vi "Exercise 10.3_Answer.vi"() -> ()   [LabVIEW 2010]
uses:
  Global 1.vi
panel:
  in  "Restart":bool
  in  "Stop":bool
  in  "Walk Request":bool
  out "Walk Sign":bool
  out "Green":bool
  out "Yellow":bool
  out "Red":bool
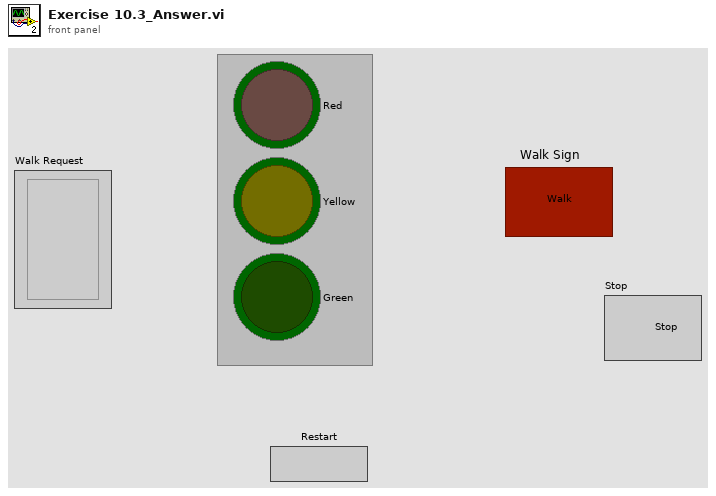
[diagram p1: front panel]
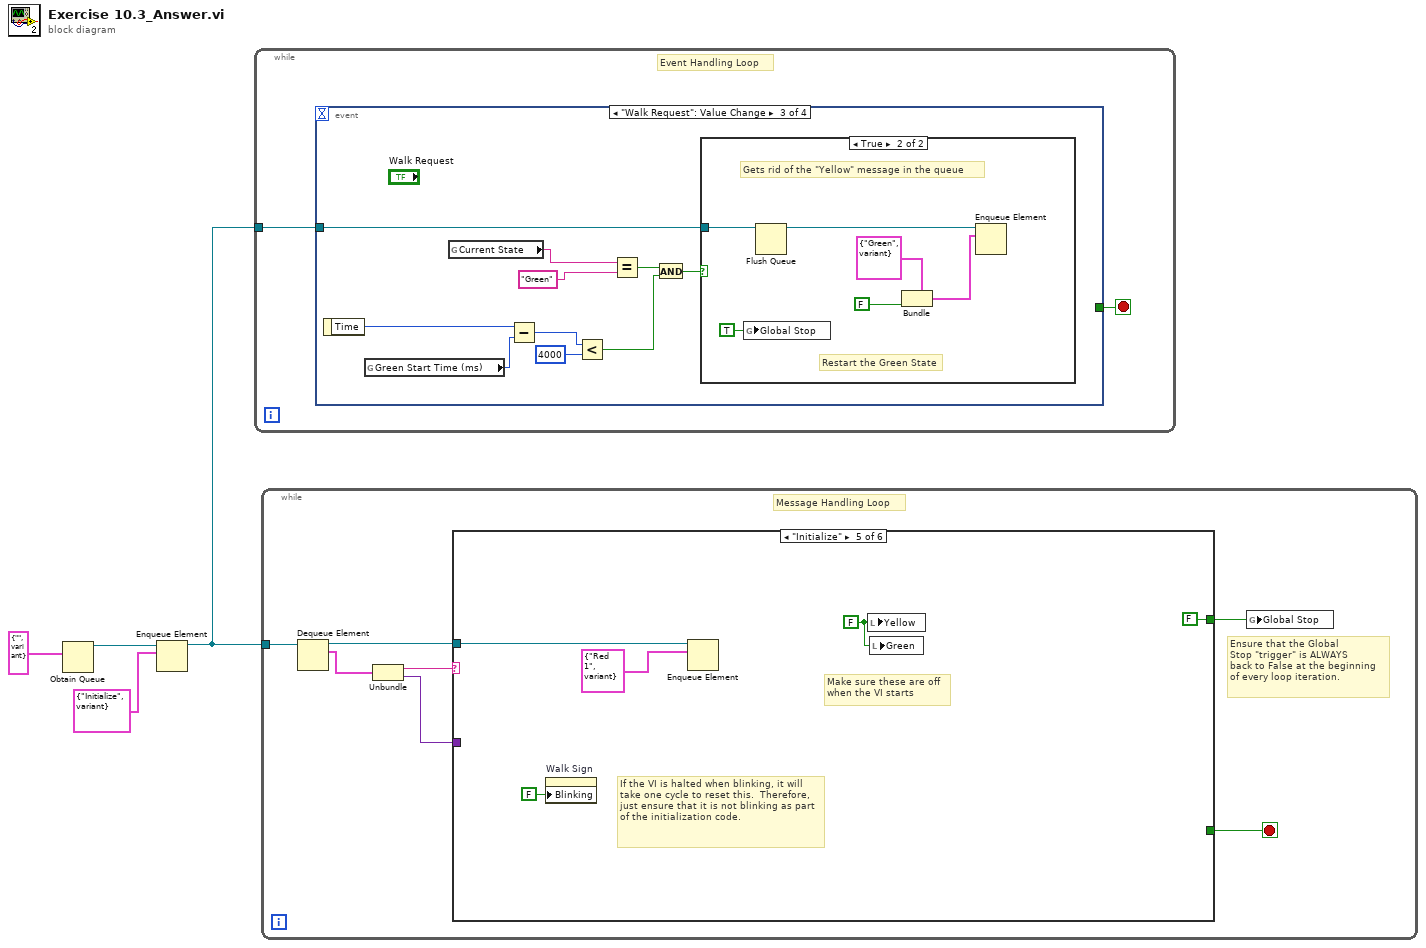
[diagram p0: block diagram]
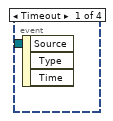
[diagram p2: hidden frame]
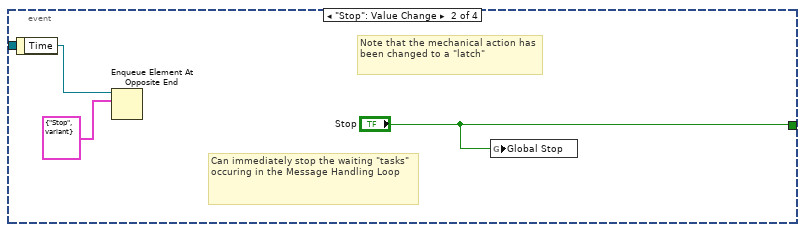
[diagram p3: hidden frame]
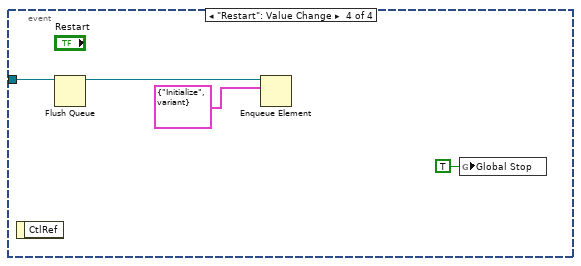
[diagram p5: hidden frame]
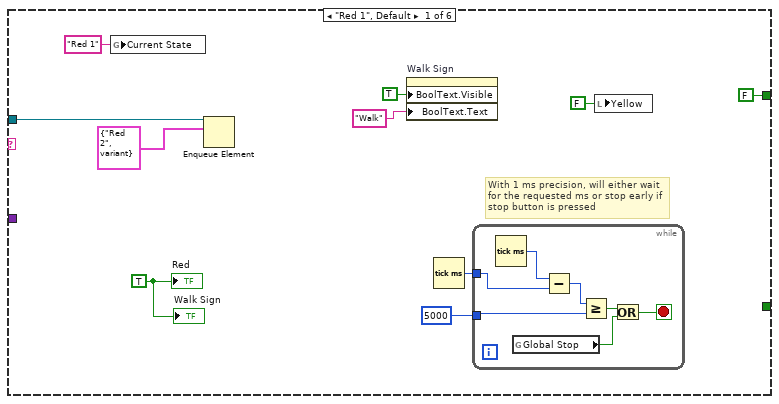
[diagram p6: hidden frame]
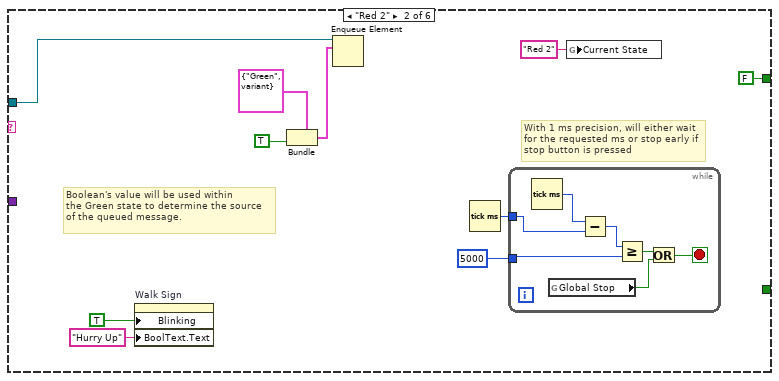
[diagram p7: hidden frame]
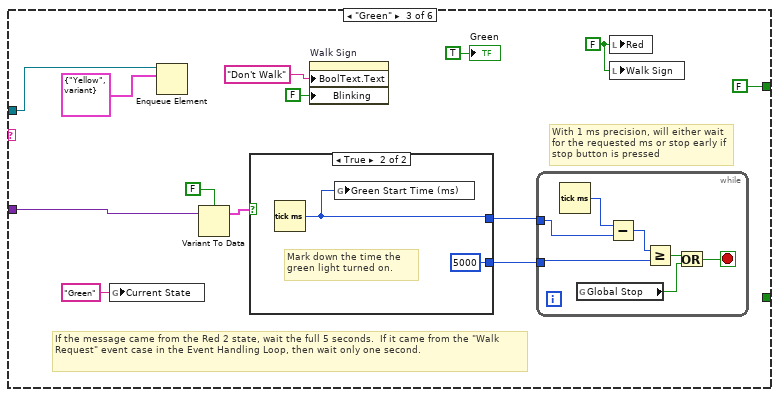
[diagram p8: hidden frame]
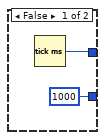
[diagram p9: hidden frame]
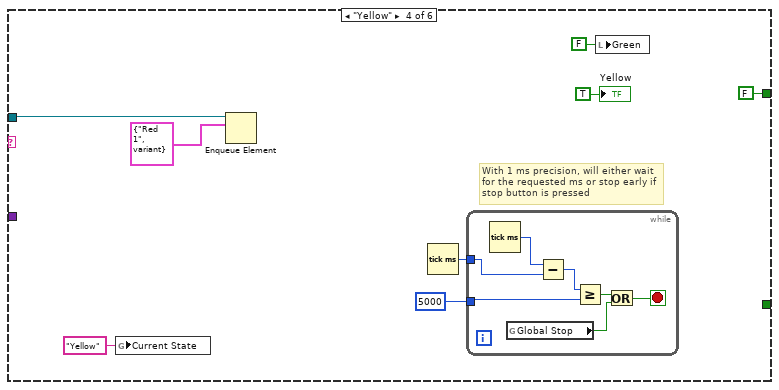
[diagram p10: hidden frame]
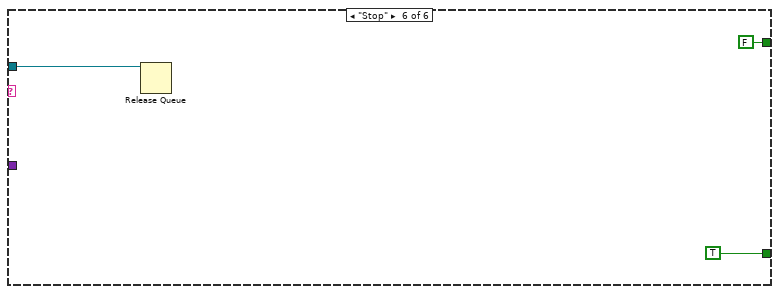
[diagram p11: hidden frame]
diagram:
  n1 = Obtain Queue(element data type=cluster{string, variant} {"", variant}) -> (queue out=w3:refnum<queue>)  [unwired: 4 in, 2 out]
  n2 = Enqueue Element(queue=w3, element=cluster{string, variant} {"Initialize", variant}) -> (queue out=w1:refnum<queue>)  [unwired: 2 in, 2 out]
  n3 = while {
    tunnel: w1 -> [w5]
    stop <- w6 stop-if-true
    # "Event Handling Loop"
    n4 = event shown="[2] \"Walk Request\": Value Change" {
      selector: _ -> [_ _ _ _]
      dyn-events: _ -> [_ _ _ _]
      timeout: _ -> [_ _ _ _]
      tunnel: [_ "Stop" _ _] -> w6
      tunnel: w5 -> [_ w8 w11 w27]
      event Timeout {
        n5 = event-data() -> ()  [unwired: 1 in, 3 out]
      }
      event "Stop": Value Change {
        # "Can immediately stop the waiting \"tasks\" occuring in the Message Handling Loop"
        # "Note that the mechanical action has been changed to a \"latch\""
        n6 = event-data() -> ()  [unwired: 1 in, 1 out]
        n7 = Enqueue Element At Opposite End(queue=w8, element=cluster{string, variant} {"Stop", variant}) -> ()  [unwired: 2 in, 3 out]
        n8 = global write "Global 1.vi" "Global Stop"("Stop") -> ()
      }
      event "Walk Request": Value Change {
        n9 = event-data() -> ("Time"=w19:u32)  [unwired: 1 in]
        n10 = global read "Global 1.vi" "Green Start Time (ms)"() -> (w18:u32)
        n11 = global read "Global 1.vi" "Current State"() -> (w16:string)
        n12 = Subtract(x=w19, y=w18) -> (x-y=w10:u32)
        n13 = Less?(x=w10, y=u32 4000) -> (x < y?=w13:bool)
        n14 = Equal?(x=w16, y="Green") -> (x = y?=w14:bool)
        n15 = And(x=w14, y=w13) -> (x .and. y?=w12:bool)
        n16 = case shown="True" w12 {
          tunnel: w11 -> [_ w24]
          frame False {
          }
          frame True {
            # "Gets rid of the \"Yellow\" message in the queue"
            # "Restart the Green State"
            n17 = global write "Global 1.vi" "Global Stop"(TRUE ("Global Stop")) -> ()
            n18 = Flush Queue(queue=w24) -> (queue out=w23:refnum<queue>)  [unwired: 1 in, 2 out]
            n19 = Bundle(cluster=cluster{string, variant} {"Green", variant} ("element"), FALSE ("Global Stop")) -> (w20:cluster{string, variant})  [unwired: 1 in]
            n20 = Enqueue Element(queue=w23, element=w20) -> ()  [unwired: 2 in, 3 out]
          }
        }
      }
      event "Restart": Value Change {
        n21 = event-data() -> ()  [unwired: 1 in, 1 out]
        n22 = Flush Queue(queue=w27) -> (queue out=w26:refnum<queue>)  [unwired: 1 in, 2 out]
        n23 = Enqueue Element(queue=w26, element=cluster{string, variant} {"Initialize", variant}) -> ()  [unwired: 2 in, 3 out]
        n24 = global write "Global 1.vi" "Global Stop"(TRUE ("Global Stop")) -> ()
      }
    }
  }
  n25 = while {
    tunnel: w1 -> [w36]
    stop <- w32 stop-if-true
    # "Ensure that the Global\nStop \"trigger\" is ALWAYS\nback to False at the beginning\nof every loop iteration."
    # "Message Handling Loop"
    n26 = Dequeue Element(queue=w36) -> (queue out=w35:refnum<queue>, element=w34:cluster{string, variant})  [unwired: 2 in, 2 out]
    n27 = Unbundle(w34) -> (w33:string, w31:variant)
    n28 = case shown="\"Initialize\"" w33 {
      tunnel: w35 -> [w41 w59 w82 w98 w112 w116]
      tunnel: [_ _ _ _ _ TRUE] -> w32
      tunnel: w31 -> [_ _ w77 _ _ _]
      tunnel: [FALSE ("Global Stop") FALSE ("Global Stop") FALSE ("Global Stop") FALSE ("Global Stop") FALSE ("Global Stop") FALSE ("Global Stop")] -> w30
      frame "Red 1", Default {
        w44 = TRUE ("Red")
        # "With 1 ms precision, will either wait for the requested ms or stop early if stop button is pressed"
        n29 = global write "Global 1.vi" "Current State"("Red 1" ("Current State")) -> ()
        n30 = Enqueue Element(queue=w41, element=cluster{string, variant} {"Red 2", variant}) -> ()  [unwired: 2 in, 3 out]
        n31 = property on="Walk Sign" class="Bool"("BoolText.Visible"=TRUE ("Boolean Text.Visible"), "BoolText.Text"="Walk" ("Boolean Text.Text")) -> ()  [unwired: 2 in, 2 out]
        n32 = Tick Count (ms)() -> (millisecond timer value=w40:u32)
        n33 = while {
          tunnel: w40 -> [w52]
          tunnel: u32 5000 ("milliseconds to wait") -> [w50]
          stop <- w48 stop-if-true
          n34 = Tick Count (ms)() -> (millisecond timer value=w53:u32)
          n35 = global read "Global 1.vi" "Global Stop"() -> (w47:bool)
          n36 = Subtract(x=w53, y=w52) -> (x-y=w51:u32)
          n37 = Greater Or Equal?(x=w51, y=w50) -> (x >= y?=w49:bool)
          n38 = Or(x=w49, y=w47) -> (x .or. y?=w48:bool)
        }
        n39 = local write "Yellow"(FALSE ("Yellow")) -> ()
        "Red" <- w44
        "Walk Sign" <- w44
      }
      frame "Red 2" {
        # "Boolean's value will be used within\nthe Green state to determine the source\nof the queued message."
        # "With 1 ms precision, will either wait for the requested ms or stop early if stop button is pressed"
        n40 = property on="Walk Sign" class="Bool"("Blinking"=TRUE, "BoolText.Text"="Hurry Up" ("Boolean Text.Text")) -> ()  [unwired: 2 in, 2 out]
        n41 = Bundle(cluster=cluster{string, variant} {"Green", variant} ("element"), TRUE) -> (w57:cluster{string, variant})  [unwired: 1 in]
        n42 = Enqueue Element(queue=w59, element=w57) -> ()  [unwired: 2 in, 3 out]
        n43 = Tick Count (ms)() -> (millisecond timer value=w61:u32)
        n44 = while {
          tunnel: w61 -> [w69]
          tunnel: u32 5000 ("milliseconds to wait") -> [w67]
          stop <- w65 stop-if-true
          n45 = Tick Count (ms)() -> (millisecond timer value=w70:u32)
          n46 = global read "Global 1.vi" "Global Stop"() -> (w64:bool)
          n47 = Subtract(x=w70, y=w69) -> (x-y=w68:u32)
          n48 = Greater Or Equal?(x=w68, y=w67) -> (x >= y?=w66:bool)
          n49 = Or(x=w66, y=w64) -> (x .or. y?=w65:bool)
        }
        n50 = global write "Global 1.vi" "Current State"("Red 2" ("Current State")) -> ()
      }
      frame "Green" {
        w80 = FALSE ("Red")
        # "If the message came from the Red 2 state, wait the full 5 seconds.  If it came from the \"Walk Request\" event case in the Event Handling Loop, then wait only one second."
        # "With 1 ms precision, will either wait for the requested ms or stop early if stop button is pressed"
        n51 = global write "Global 1.vi" "Current State"("Green" ("Current State")) -> ()
        n52 = Enqueue Element(queue=w82, element=cluster{string, variant} {"Yellow", variant}) -> ()  [unwired: 2 in, 3 out]
        n53 = Variant To Data(Variant=w77, type=FALSE) -> (data=w72:cluster{})  [unwired: 1 in, 1 out]
        n54 = case shown="True" w72 {
          tunnel: [u32 1000 ("milliseconds to wait") u32 5000 ("milliseconds to wait")] -> w76
          tunnel: [w85 w86] -> w75
          frame False {
            n55 = Tick Count (ms)() -> (millisecond timer value=w85:u32)
          }
          frame True {
            # "Mark down the time the \ngreen light turned on."
            n56 = Tick Count (ms)() -> (millisecond timer value=w86:u32)
            n57 = global write "Global 1.vi" "Green Start Time (ms)"(w86) -> ()
          }
        }
        n58 = property on="Walk Sign" class="Bool"("BoolText.Text"="Don't Walk" ("Boolean Text.Text"), "Blinking"=FALSE) -> ()  [unwired: 2 in, 2 out]
        n59 = while {
          tunnel: w75 -> [w93]
          tunnel: w76 -> [w91]
          stop <- w89 stop-if-true
          n60 = Tick Count (ms)() -> (millisecond timer value=w94:u32)
          n61 = global read "Global 1.vi" "Global Stop"() -> (w88:bool)
          n62 = Subtract(x=w94, y=w93) -> (x-y=w92:u32)
          n63 = Greater Or Equal?(x=w92, y=w91) -> (x >= y?=w90:bool)
          n64 = Or(x=w90, y=w88) -> (x .or. y?=w89:bool)
        }
        n65 = local write "Red"(w80) -> ()
        n66 = local write "Walk Sign"(w80) -> ()
        "Green" <- TRUE ("Green")
      }
      frame "Yellow" {
        # "With 1 ms precision, will either wait for the requested ms or stop early if stop button is pressed"
        n67 = global write "Global 1.vi" "Current State"("Yellow" ("Current State")) -> ()
        n68 = Enqueue Element(queue=w98, element=cluster{string, variant} {"Red 1", variant}) -> ()  [unwired: 2 in, 3 out]
        n69 = Tick Count (ms)() -> (millisecond timer value=w97:u32)
        n70 = while {
          tunnel: w97 -> [w108]
          tunnel: u32 5000 ("milliseconds to wait") -> [w106]
          stop <- w104 stop-if-true
          n71 = Tick Count (ms)() -> (millisecond timer value=w109:u32)
          n72 = global read "Global 1.vi" "Global Stop"() -> (w103:bool)
          n73 = Subtract(x=w109, y=w108) -> (x-y=w107:u32)
          n74 = Greater Or Equal?(x=w107, y=w106) -> (x >= y?=w105:bool)
          n75 = Or(x=w105, y=w103) -> (x .or. y?=w104:bool)
        }
        n76 = local write "Green"(FALSE ("Green")) -> ()
        "Yellow" <- TRUE ("Yellow")
      }
      frame "Initialize" {
        w114 = FALSE ("Yellow")
        # "If the VI is halted when blinking, it will take one cycle to reset this.  Therefore, just ensure that it is not blinking as part of the initialization code."
        # "Make sure these are off\nwhen the VI starts"
        n77 = property on="Walk Sign" class="Bool"("Blinking"=FALSE) -> ()  [unwired: 2 in, 2 out]
        n78 = Enqueue Element(queue=w112, element=cluster{string, variant} {"Red 1", variant}) -> ()  [unwired: 2 in, 3 out]
        n79 = local write "Yellow"(w114) -> ()
        n80 = local write "Green"(w114) -> ()
      }
      frame "Stop" {
        n81 = Release Queue(queue=w116) -> ()  [unwired: 2 in, 3 out]
      }
    }
    n82 = global write "Global 1.vi" "Global Stop"(w30) -> ()
  }
